vi "ReverseSplinePath.vi"(0 "original":T2[](array[typedef]), 1 "path":T1[](array[typedef])=[{"x"=12.0, "y"=150.0, "angle"=0.0}, {"x"=24.0, "y"=150.0, "angle"=0.0}, {"x"=175.0, "y"=275.0, "angle"=0.0}, {"x"=235.0, "y"=200.0, "angle"=90.0}, {"x"=235.0, "y"=125.0, "angle"=90.0}, {"x"=290.0, "y"=65.0, "angle"=0.0}], 5 "left":T2[](array[typedef]), 7 "right":T2[](array[typedef]), 11 "error in (no error)":errorcluster) -> (4 "original_out":T2[](array[typedef]), 6 "left_out":T2[](array[typedef]), 8 "right_out":T2[](array[typedef]), 14 "Inverted":bool, 15 "error out":errorcluster)   [LabVIEW 2018]
uses:
  Pathfinder/Pathfinder-LabVIEW/Pathfinder-Lib/VIs/Segment.ctl
  Pathfinder/Pathfinder-LabVIEW/Pathfinder-Lib/VIs/Waypoint.ctl
  3a6ebb16-e35f-4c6d-b4d5-97db8c5ad900.vi
  672ebdab-1f90-49c9-a55e-2541e44076d6.vi
  c0a805b6-889d-45e9-80d3-6abaa639b3d2.vi
  019bdce3-3ff9-42a6-8bc7-9cfecdf4b622.vi
  ArgosLib/ArgosLib.lvlib
  Pathfinder/Pathfinder-LabVIEW/Pathfinder-Lib/Pathfinder.lvlib
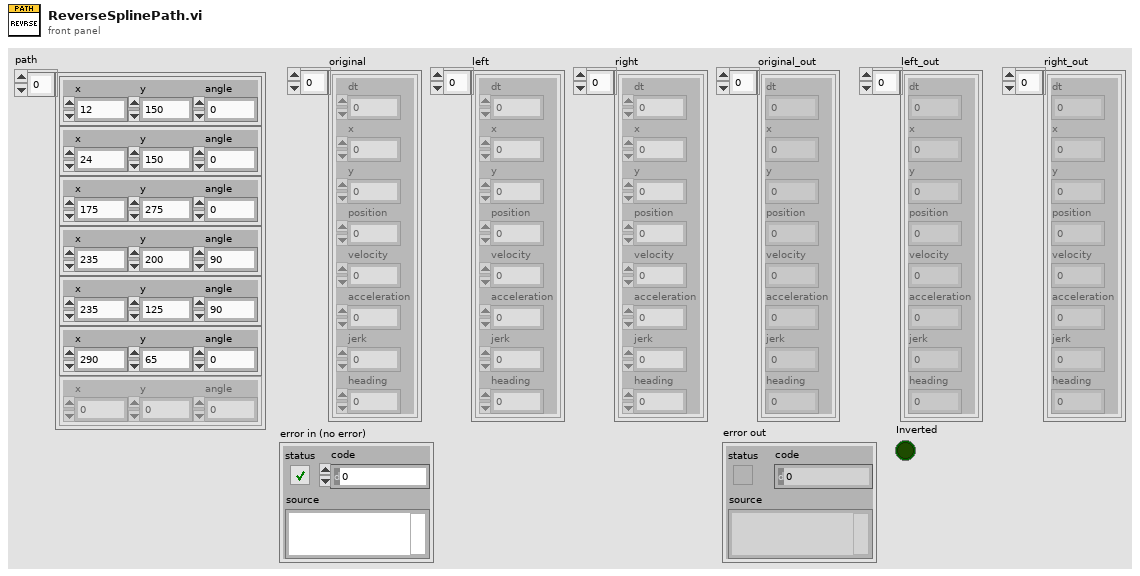
[diagram p1: front panel]
types:
  T1 = typedef "Pathfinder.lvlib/Waypoint.ctl" = cluster{"x":dbl, "y":dbl, "angle":dbl}
  T2 = typedef "Pathfinder.lvlib/Segment.ctl" = cluster{"dt":dbl, "x":dbl, "y":dbl, "position":dbl, "velocity":dbl, "acceleration":dbl, "jerk":dbl, "heading":dbl}
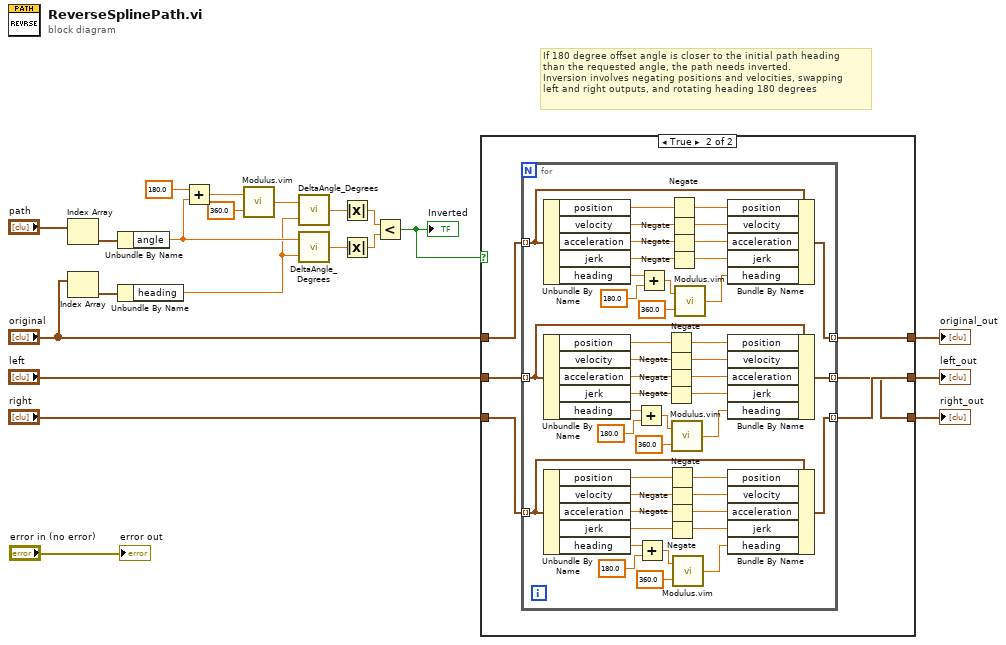
[diagram p0: block diagram]
diagram:
  # "If 180 degree offset angle is closer to the initial path heading\nthan the requested angle, the path needs inverted.\nInversion involves negating positions and velocities, swapping\nleft and right outputs, and rotating heading 180 degrees"
  n1 = Index Array(array="path") -> (element=w19:T1)  [unwired: 1 in]
  n2 = Index Array(array="original") -> (element=w18:T2)  [unwired: 1 in]
  n3 = Unbundle By Name(w19) -> ("angle"=w17:dbl)
  n4 = Unbundle By Name(w18) -> ("heading"=w15:dbl)
  n5 = Add(x=180.0, y=w17) -> (x+y=w10:dbl)
  n6 = call "Modulus.vim"("y"=360.0, "x"=w10) -> ("x%y"=w9:dbl)
  n7 = call "DeltaAngle_Degrees.vi"("EndAngle (deg)"=w15, "StartAngle (deg)"=w9) -> ("DeltaAngle (deg)"=w14:dbl)
  n8 = call "DeltaAngle_Degrees.vi"("EndAngle (deg)"=w15, "StartAngle (deg)"=w17) -> ("DeltaAngle (deg)"=w13:dbl)
  n9 = Absolute Value(x=w14) -> (abs(x)=w12:dbl)
  n10 = Absolute Value(x=w13) -> (abs(x)=w11:dbl)
  n11 = Less?(x=w12, y=w11) -> (x < y?=w7:bool)
  "Inverted" <- w7
  n12 = case shown="True" w7 {
    tunnel: "original" -> [w24 w28]
    tunnel: "left" -> [w23 w29]
    tunnel: "right" -> [w22 w30]
    tunnel: [w24 w27] -> w1
    tunnel: [w23 w26] -> w2
    tunnel: [w22 w25] -> w3
    frame False {
    }
    frame True {
      n13 = for {
        tunnel: w30 -> [w34] mode=indexing
        tunnel: w29 -> [w35] mode=indexing
        tunnel: w28 -> [w71] mode=indexing
        tunnel: [w31] -> w27 mode=indexing
        tunnel: [w33] -> w25 mode=indexing
        tunnel: [w32] -> w26 mode=indexing
        n14 = Unbundle By Name(w71) -> ("position"=w66:dbl, "velocity"=w67:dbl, "acceleration"=w68:dbl, "jerk"=w69:dbl, "heading"=w72:dbl)
        n15 = Unbundle By Name(w35) -> ("position"=w57:dbl, "velocity"=w56:dbl, "acceleration"=w55:dbl, "jerk"=w54:dbl, "heading"=w52:dbl)
        n16 = Unbundle By Name(w34) -> ("position"=w40:dbl, "velocity"=w41:dbl, "acceleration"=w42:dbl, "jerk"=w43:dbl, "heading"=w45:dbl)
        n17 = Add(x=w52, y=180.0) -> (x+y=w50:dbl)
        n18 = Add(x=w45, y=180.0) -> (x+y=w47:dbl)
        n19 = Add(x=w72, y=180.0) -> (x+y=w74:dbl)
        n20 = Negate(x=w57) -> (-x=w58:dbl)
        n21 = Negate(x=w56) -> (-x=w59:dbl)
        n22 = Negate(x=w55) -> (-x=w60:dbl)
        n23 = Negate(x=w54) -> (-x=w61:dbl)
        n24 = Negate(x=w40) -> (-x=w39:dbl)
        n25 = Negate(x=w41) -> (-x=w38:dbl)
        n26 = Negate(x=w42) -> (-x=w37:dbl)
        n27 = Negate(x=w43) -> (-x=w36:dbl)
        n28 = Negate(x=w66) -> (-x=w65:dbl)
        n29 = Negate(x=w67) -> (-x=w64:dbl)
        n30 = Negate(x=w68) -> (-x=w63:dbl)
        n31 = Negate(x=w69) -> (-x=w62:dbl)
        n32 = call "Modulus.vim"("y"=360.0, "x"=w50) -> ("x%y"=w53:dbl)
        n33 = call "Modulus.vim"("y"=360.0, "x"=w47) -> ("x%y"=w44:dbl)
        n34 = call "Modulus.vim"("y"=360.0, "x"=w74) -> ("x%y"=w70:dbl)
        n35 = Bundle By Name(cluster=w71, "position"=w65, "velocity"=w64, "acceleration"=w63, "jerk"=w62, "heading"=w70) -> (w31:T2)
        n36 = Bundle By Name(cluster=w35, "position"=w58, "velocity"=w59, "acceleration"=w60, "jerk"=w61, "heading"=w53) -> (w33:T2)
        n37 = Bundle By Name(cluster=w34, "position"=w39, "velocity"=w38, "acceleration"=w37, "jerk"=w36, "heading"=w44) -> (w32:T2)
      }
    }
  }
  "original_out" <- w1
  "left_out" <- w2
  "right_out" <- w3
  "error out" <- "error in (no error)"
